vi "Send Error to Notebook.vi"(8 "error in (no error)":errorcluster, 9 "Verbose Error Messages (T)":bool=TRUE, 10 "State Machine Case Error Source":string, 11 "Notebook Q":refnum<queue>) -> (0 "Error Out":errorcluster)   [LabVIEW 2019, in "Notebook.lvlib"]
uses:
  Notebook.lvlib
  Notebook Action Q Element.ctl
  Notebook Action List.ctl
  Sound/System Sounds List.ctl
  Notebook Saved Global.vi
  Rich Text Box/Rich Text Box.lvlib
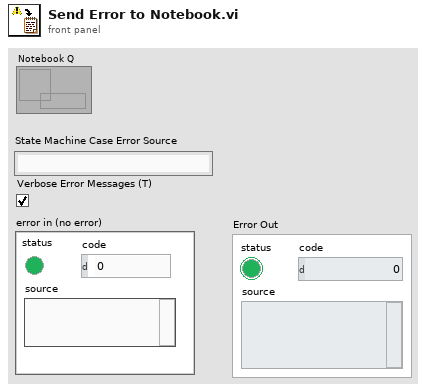
[diagram p1: front panel]
types:
  T1 = typedef "System Sounds List.ctl" = enum16{"Alarm01", "Alarm02", "Alarm03", "Alarm04", "Alarm05", "Alarm06", "Alarm07", "Alarm08", "Alarm09", "Alarm10", "chimes", "chord", "ding", "notify", "recycle", "Ring01", "Ring02", "Ring03", "Ring04", "Ring05", "Ring06", "Ring07", "Ring08", "Ring09", "Ring10", "ringout", "Speech Off", "Speech On", "Speech Sleep", "tada", "Windows Background", "Windows Balloon", "Windows Battery Critical", "Windows Battery Low", "Windows Critical Stop", "Windows Default", "Windows Ding", "Windows Error", "Windows Exclamation", "Windows Feed Discovered", "Windows Foreground", "Windows Hardware Fail", "Windows Hardware Insert", "Windows Hardware Remove", "Windows Information Bar", "Windows Logoff Sound", "Windows Logon", "Windows Menu Command", "Windows Message Nudge", "Windows Minimize", "Windows Navigation Start", "Windows Notify Calendar", "Windows Notify Email", "Windows Notify Messaging", "Windows Notify System Generic", "Windows Notify", "Windows Pop-up Blocked", "Windows Print complete", "Windows Proximity Connection", "Windows Proximity Notification", "Windows Recycle", "Windows Restore", "Windows Ringin", "Windows Ringout", "Windows Shutdown", "Windows Startup", "Windows Unlock", "Windows User Account Control"}
  T2 = typedef "Rich Text Box.lvlib/Text Formatting.ctl" = cluster{"Font":string, "Text Color":T3, "Text Background Color":T3, "Text Style":enum16{"Regular", "Bold", "Italic", "Underline", "Strikeout"}, "Font Size (Points)":dbl, "Text Alignment":i32}
  T3 = typedef "Rich Text Box.lvlib/Text Colors.ctl" = enum16{"Unchanged", "Black", "Blue", "Brown", "Gray", "Green", "Orange", "Pink", "Red", "White"}
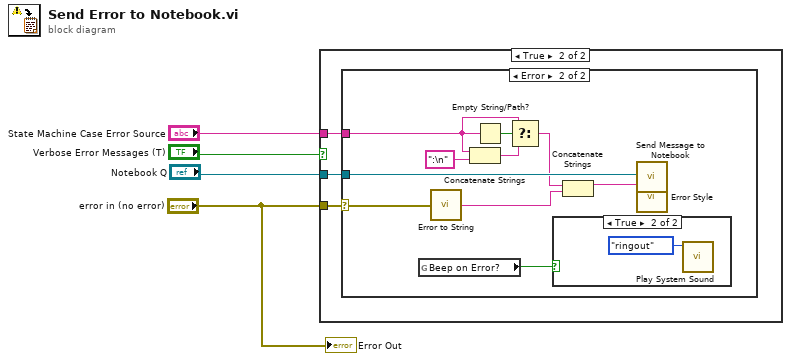
[diagram p0: block diagram]
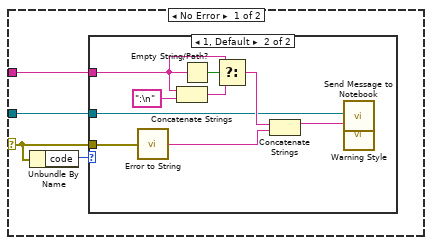
[diagram p3: hidden frame]
diagram:
  n1 = case shown="True" "Verbose Error Messages (T)" {
    tunnel: "Notebook Q" -> [_ w7]
    tunnel: "State Machine Case Error Source" -> [_ w6]
    tunnel: "error in (no error)" -> [_ w5]
    frame False {
    }
    frame True {
      n2 = case shown="Error" w5 {
        selector: w5 -> [w9 w30]
        tunnel: w7 -> [w11 w32]
        tunnel: w6 -> [w8 w31]
        frame No Error {
          n3 = Unbundle By Name(w9) -> ("code"=w10:i32)
          n4 = case shown="1, Default" w10 {
            tunnel: w11 -> [_ w15]
            tunnel: w9 -> [_ w14]
            tunnel: w8 -> [_ w13]
            frame 0 {
            }
            frame 1, Default {
              n5 = call "Error to String.vi"("error in (no error)"=w14) -> ("message"=w16:string)  [unwired: 8 in]
              n6 = Concatenate Strings(w13, ":\n" ("string")) -> (w17:string)
              n7 = Empty String/Path?(string/path=w13) -> (empty?=w20:bool)
              n8 = Select(t=w13, s=w20, f=w17) -> (s? t:f=w19:string)
              n9 = Concatenate Strings(w19, w16) -> (w21:string)
              n10 = call "Warning Style.vi"() -> ("Error Formatting"=w12:T2)
              n11 = call "Send Message to Notebook.vi"("Notebook Queue"=w15, "Message"=w21, "Text Formatting"=w12) -> ()  [unwired: 16 in, 1 out]
            }
          }
        }
        frame Error {
          n12 = global read "Notebook Saved Global.vi" "Beep on Error?"() -> (w22:bool)
          n13 = call "Error to String.vi"("error in (no error)"=w30) -> ("message"=w24:string)  [unwired: 8 in]
          n14 = Concatenate Strings(w31, ":\n" ("string")) -> (w25:string)
          n15 = Empty String/Path?(string/path=w31) -> (empty?=w28:bool)
          n16 = Select(t=w31, s=w28, f=w25) -> (s? t:f=w27:string)
          n17 = case shown="True" w22 {
            frame False {
            }
            frame True {
              n18 = call "Play System Sound.vi"("Windows Sound"=System_Sounds_List."ringout") -> ()  [unwired: 10 in, 1 out]
            }
          }
          n19 = Concatenate Strings(w27, w24) -> (w29:string)
          n20 = call "Error Style.vi"() -> ("Error Formatting"=w23:T2)
          n21 = call "Send Message to Notebook.vi"("Notebook Queue"=w32, "Message"=w29, "Text Formatting"=w23) -> ()  [unwired: 16 in, 1 out]
        }
      }
    }
  }
  "Error Out" <- "error in (no error)"
